vi "zifuchuanchaifentest1.vi"() -> ()   [LabVIEW 2020]
panel:
  out "连接的字符串 3":string
  in  "位置环pid：\n     设定位置3 2":i32=1000
  out "字符串 3":string
  out "十六进制整型字符串 3":string
  in  "位置环pid：\n     设定位置3":i32=1000
  out "连接的字符串 2":string
  out "循环次数":i32
  out "连接的字符串":string
  out "字符串 2":string
  out "十六进制整型字符串 2":string
  in  "位置环pid：\n     设定位置 2":i32=1000
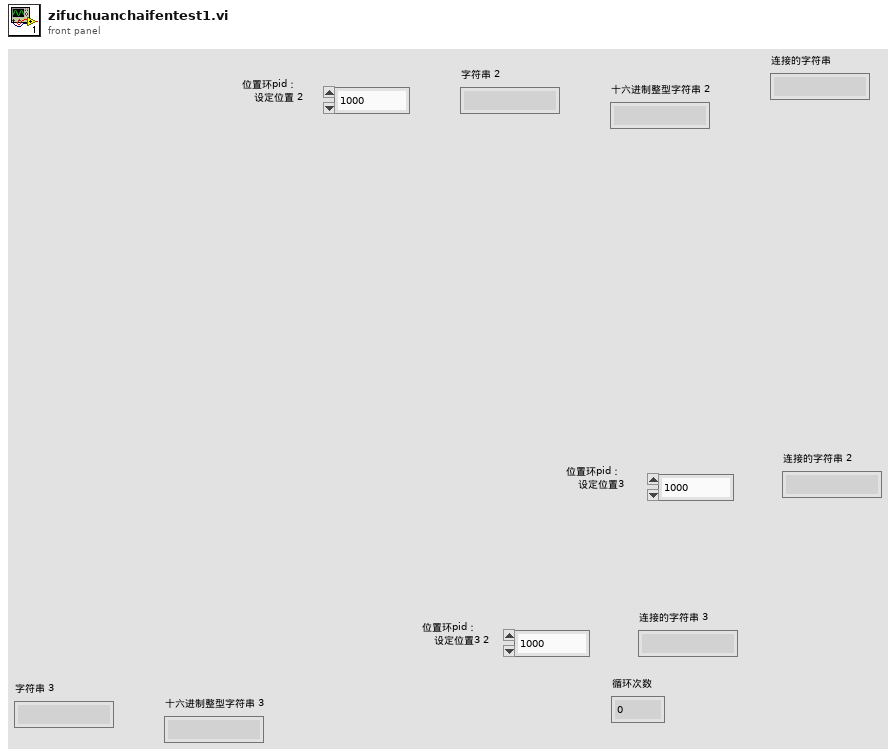
[diagram p1: front panel]
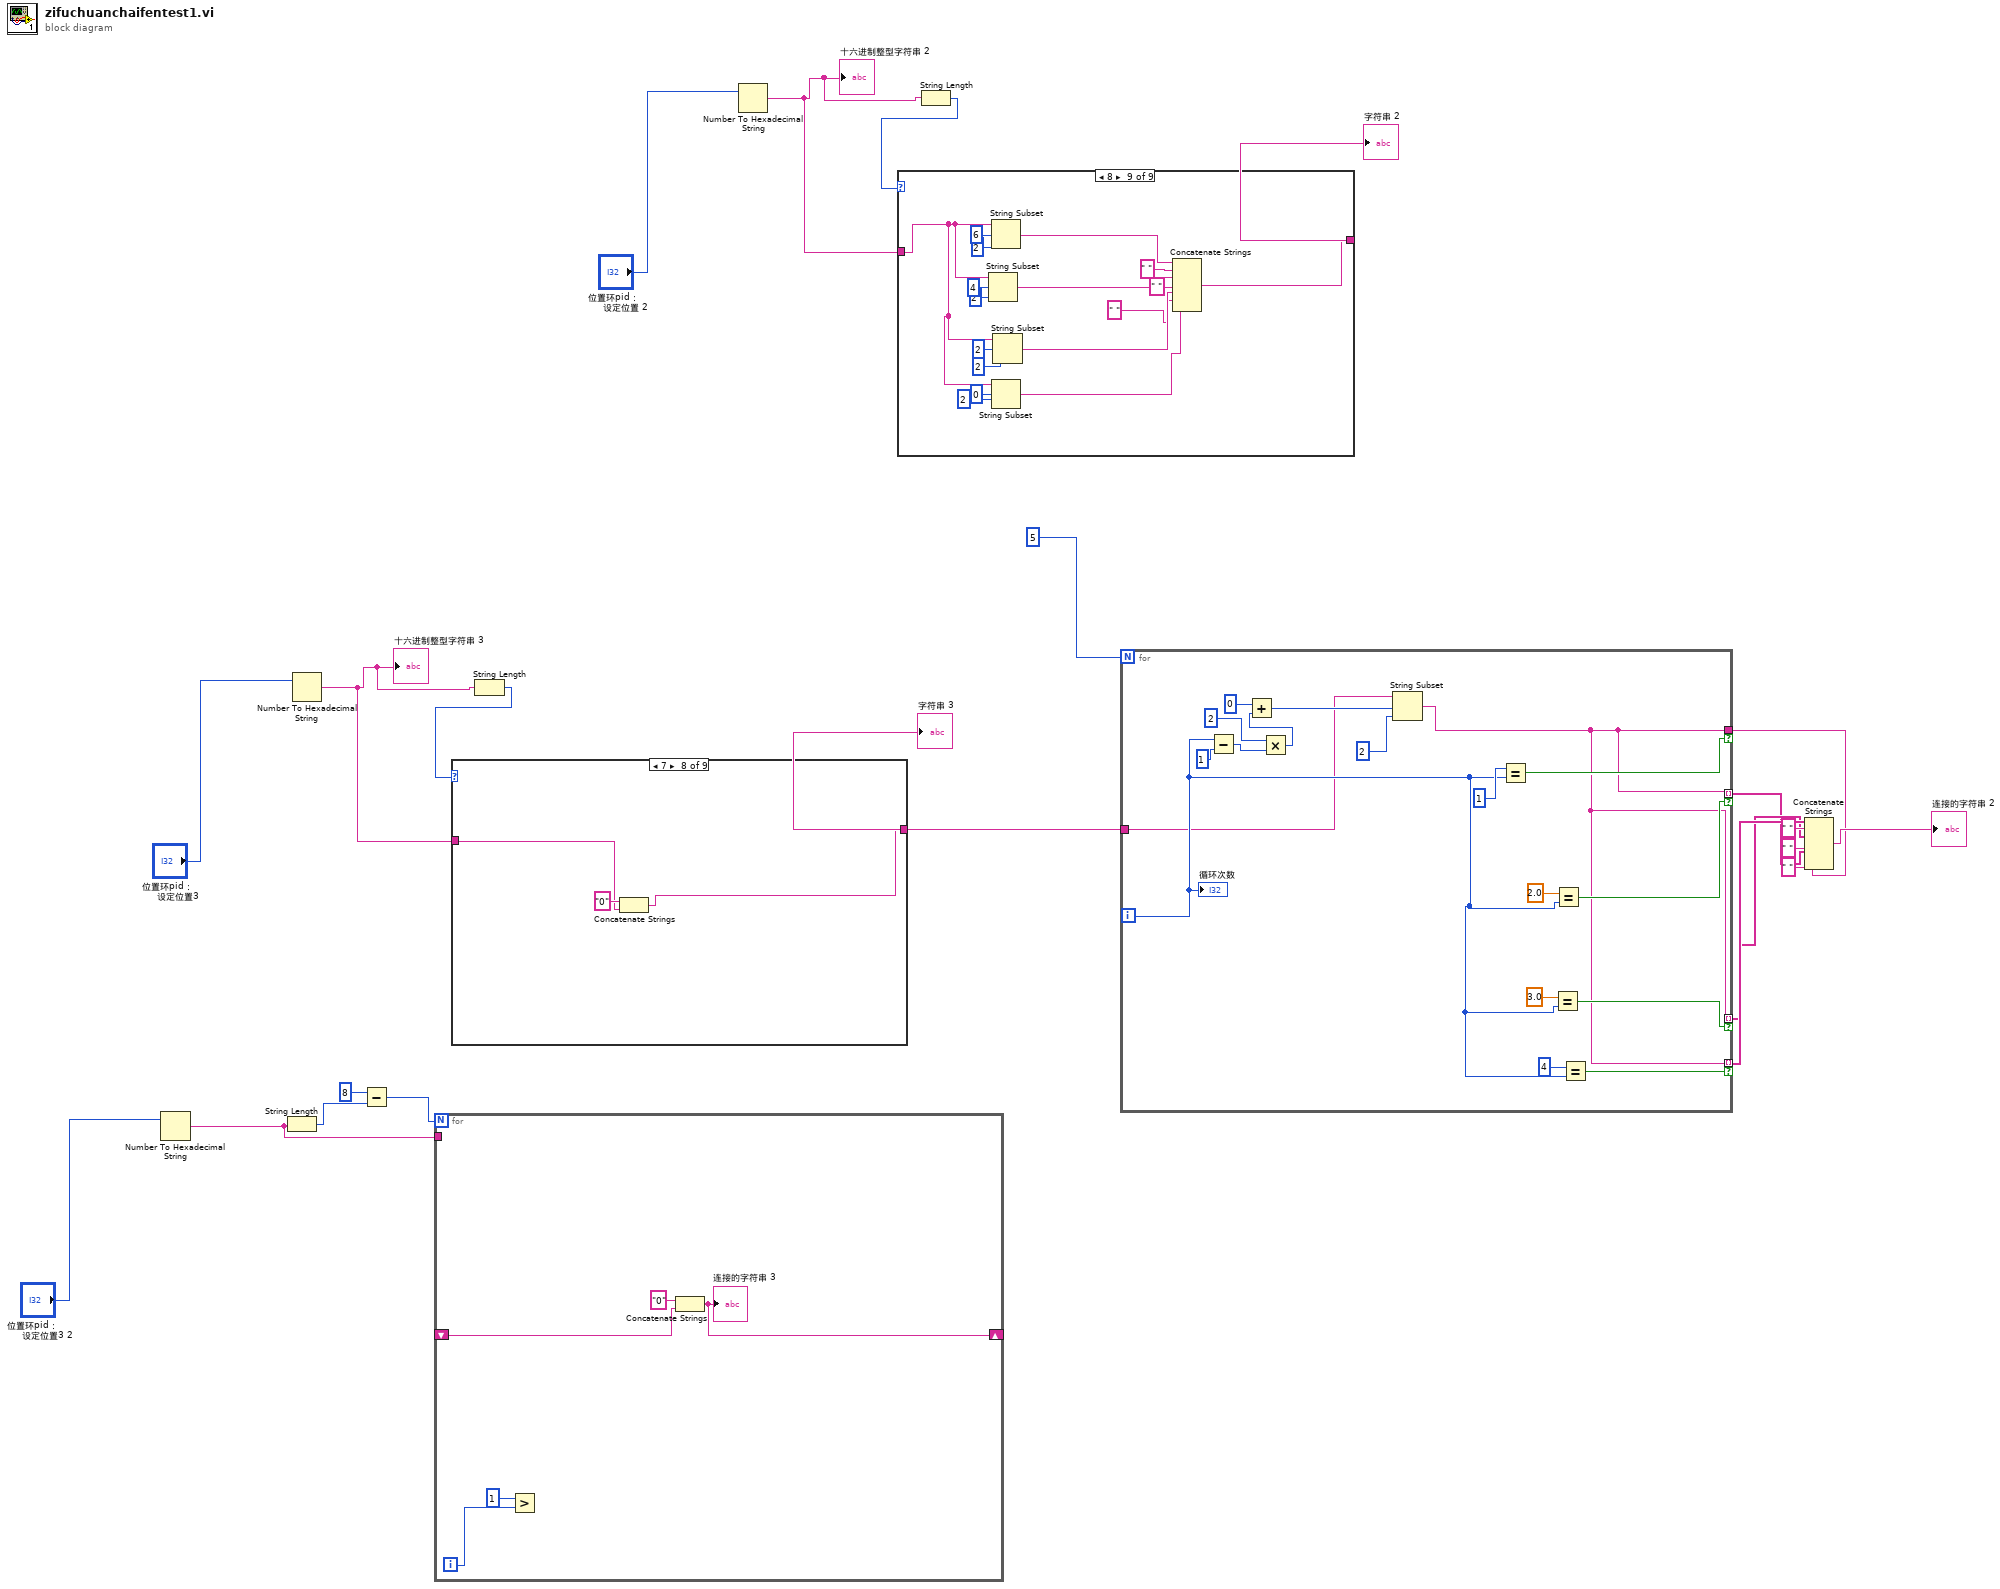
[diagram p0: block diagram]
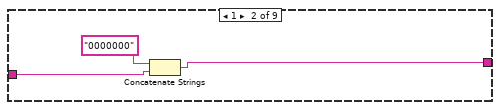
[diagram p3: hidden frame]
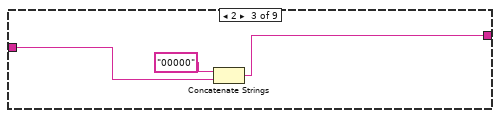
[diagram p4: hidden frame]
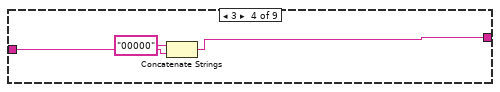
[diagram p5: hidden frame]
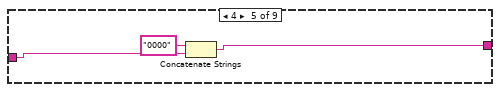
[diagram p6: hidden frame]
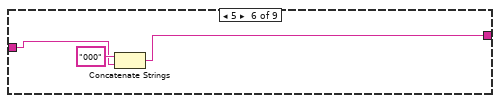
[diagram p7: hidden frame]
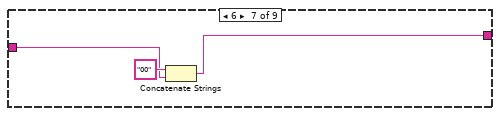
[diagram p8: hidden frame]
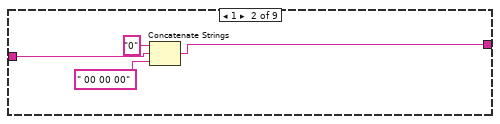
[diagram p11: hidden frame]
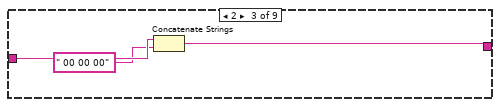
[diagram p12: hidden frame]
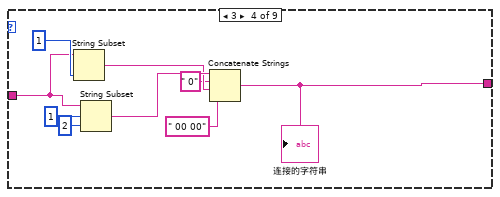
[diagram p13: hidden frame]
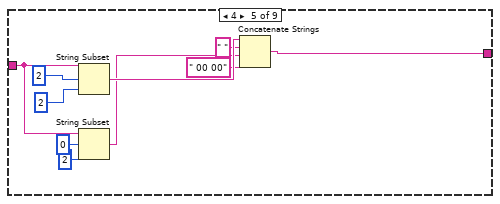
[diagram p14: hidden frame]
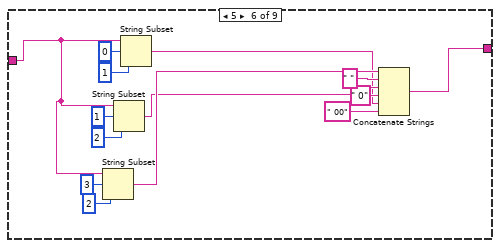
[diagram p15: hidden frame]
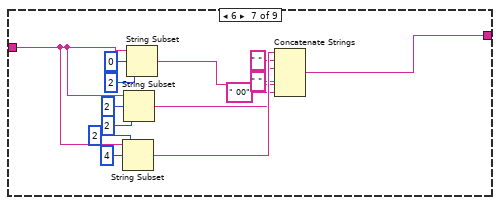
[diagram p16: hidden frame]
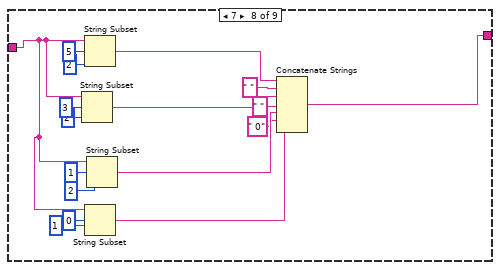
[diagram p17: hidden frame]
diagram:
  n1 = Number To Hexadecimal String(2:"位置环pid：\n     设定位置3 2") -> (0:w4:string)  [unwired: 1 in]
  n2 = String Length(string=w4) -> (length=w3:i32)
  n3 = Number To Hexadecimal String(2:"位置环pid：\n     设定位置3") -> (0:w15:string)  [unwired: 1 in]
  "十六进制整型字符串 3" <- w15
  n4 = Subtract(x=8, y=w3) -> (x-y=w1:i32)
  n5 = for {
    N: w1 -> [_]
    tunnel: w4 -> [_]
    shift-right: [w26] -> _
    shift-left: _ -> [w25]
    i -> [w24]
    n6 = Greater?(x=1, y=w24) -> ()  [unwired: 1 out]
    n7 = Concatenate Strings("0" ("字符串"), w25) -> (w26:string)
    "连接的字符串 3" <- w26
  }
  n8 = String Length(string=w15) -> (length=w16:i32)
  n9 = case shown="7" w16 {
    tunnel: w15 -> [w28 w30 w33 w37 w40 w42 w45 w48 w50]
    tunnel: [w28 w29 w32 w36 w38 w41 w44 w47 w50] -> w14
    frame 0, Default {
    }
    frame 1 {
      n10 = Concatenate Strings("0000000" ("字符串"), w30) -> (w29:string)
    }
    frame 2 {
      n11 = Concatenate Strings("00000" ("字符串"), w33) -> (w32:string)
    }
    frame 3 {
      n12 = Concatenate Strings("00000" ("字符串"), w37) -> (w36:string)
    }
    frame 4 {
      n13 = Concatenate Strings("0000" ("字符串"), w40) -> (w38:string)
    }
    frame 5 {
      n14 = Concatenate Strings("000" ("字符串"), w42) -> (w41:string)
    }
    frame 6 {
      n15 = Concatenate Strings("00" ("字符串"), w45) -> (w44:string)
    }
    frame 7 {
      n16 = Concatenate Strings("0" ("字符串"), w48) -> (w47:string)
    }
    frame 8 {
    }
  }
  "字符串 3" <- w14
  n17 = Number To Hexadecimal String(2:"位置环pid：\n     设定位置 2") -> (0:w19:string)  [unwired: 1 in]
  "十六进制整型字符串 2" <- w19
  n18 = String Length(string=w19) -> (length=w20:i32)
  n19 = case shown="8" w20 {
    tunnel: w19 -> [w51 w54 w57 w64 w73 w87 w100 w116 w126]
    tunnel: [w51 w53 w58 w59 w77 w84 w105 w106 w125] -> w21
    frame 0, Default {
    }
    frame 1 {
      n20 = Concatenate Strings("0" ("字符串"), w54, " 00 00 00" ("字符串")) -> (w53:string)
    }
    frame 2 {
      n21 = Concatenate Strings(w57, " 00 00 00" ("字符串")) -> (w58:string)
    }
    frame 3 {
      n22 = String Subset(string=w64, length (rest)=1 ("长度（剩余）")) -> (substring=w62:string)  [unwired: 1 in]
      n23 = String Subset(string=w64, offset (0)=1 ("偏移量(0)"), length (rest)=2 ("长度（剩余）")) -> (substring=w63:string)
      n24 = Concatenate Strings(w63, " 0" ("字符串"), w62, " 00 00" ("字符串")) -> (w59:string)
      "连接的字符串" <- w59
    }
    frame 4 {
      n25 = String Subset(string=w73, offset (0)=2 ("偏移量(0)"), length (rest)=2 ("长度（剩余）")) -> (substring=w74:string)
      n26 = String Subset(string=w73, offset (0)=0 ("偏移量(0)"), length (rest)=2 ("长度（剩余）")) -> (substring=w69:string)
      n27 = Concatenate Strings(w74, " " ("字符串"), w69, " 00 00" ("字符串")) -> (w77:string)
    }
    frame 5 {
      n28 = String Subset(string=w87, offset (0)=3 ("偏移量(0)"), length (rest)=2 ("长度（剩余）")) -> (substring=w83:string)
      n29 = String Subset(string=w87, offset (0)=1 ("偏移量(0)"), length (rest)=2 ("长度（剩余）")) -> (substring=w81:string)
      n30 = String Subset(string=w87, offset (0)=0 ("偏移量(0)"), length (rest)=1 ("长度（剩余）")) -> (substring=w79:string)
      n31 = Concatenate Strings(w83, " " ("字符串"), w81, " 0" ("字符串"), w79, " 00" ("字符串")) -> (w84:string)
    }
    frame 6 {
      n32 = String Subset(string=w100, offset (0)=4 ("偏移量(0)"), length (rest)=2 ("长度（剩余）")) -> (substring=w97:string)
      n33 = String Subset(string=w100, offset (0)=2 ("偏移量(0)"), length (rest)=2 ("长度（剩余）")) -> (substring=w95:string)
      n34 = String Subset(string=w100, offset (0)=0 ("偏移量(0)"), length (rest)=2 ("长度（剩余）")) -> (substring=w93:string)
      n35 = Concatenate Strings(w97, " " ("字符串"), w95, " " ("字符串"), w93, " 00" ("字符串")) -> (w105:string)
    }
    frame 7 {
      n36 = String Subset(string=w116, offset (0)=3 ("偏移量(0)"), length (rest)=2 ("长度（剩余）")) -> (substring=w111:string)
      n37 = String Subset(string=w116, offset (0)=5 ("偏移量(0)"), length (rest)=2 ("长度（剩余）")) -> (substring=w113:string)
      n38 = String Subset(string=w116, offset (0)=0 ("偏移量(0)"), length (rest)=1 ("长度（剩余）")) -> (substring=w107:string)
      n39 = String Subset(string=w116, offset (0)=1 ("偏移量(0)"), length (rest)=2 ("长度（剩余）")) -> (substring=w109:string)
      n40 = Concatenate Strings(w113, " " ("字符串"), w111, " " ("字符串"), w109, " 0" ("字符串"), w107) -> (w106:string)
    }
    frame 8 {
      n41 = String Subset(string=w126, offset (0)=4 ("偏移量(0)"), length (rest)=2 ("长度（剩余）")) -> (substring=w129:string)
      n42 = String Subset(string=w126, offset (0)=6 ("偏移量(0)"), length (rest)=2 ("长度（剩余）")) -> (substring=w131:string)
      n43 = String Subset(string=w126, offset (0)=0 ("偏移量(0)"), length (rest)=2 ("长度（剩余）")) -> (substring=w123:string)
      n44 = String Subset(string=w126, offset (0)=2 ("偏移量(0)"), length (rest)=2 ("长度（剩余）")) -> (substring=w127:string)
      n45 = Concatenate Strings(w131, " " ("字符串"), w129, " " ("字符串"), w127, " " ("字符串"), w123) -> (w125:string)
    }
  }
  "字符串 2" <- w21
  n46 = for {
    N: 5 -> [_]
    tunnel: [w142] -> w6 if=w154
    tunnel: [w142] -> w9 mode=indexing if=w152
    tunnel: [w142] -> w10 mode=indexing if=w150
    tunnel: [w142] -> w13 mode=indexing if=w141
    tunnel: w14 -> [w140]
    i -> [w144]
    n47 = Subtract(x=w144, y=1) -> (x-y=w148:i32)
    n48 = Multiply(x=2, y=w148) -> (x*y=w146:i32)
    n49 = Add(x=0, y=w146) -> (x+y=w157:i32)
    n50 = String Subset(string=w140, offset (0)=w157, length (rest)=2 ("长度（剩余）")) -> (substring=w142:string)
    n51 = Equal?(x=1, y=w144) -> (x = y?=w154:bool)
    n52 = Equal?(x=3.0, y=w144) -> (x = y?=w150:bool)
    n53 = Equal?(x=2.0, y=w144) -> (x = y?=w152:bool)
    n54 = Equal?(x=4, y=w144) -> (x = y?=w141:bool)
    "循环次数" <- w144
  }
  n55 = Concatenate Strings(w13, " " ("字符串"), w10, " " ("字符串"), w9, " " ("字符串"), w6) -> (→"连接的字符串 2":string)
